vi "SectorOverlay.vi"(0 "Min z":dbl format="%.2f", 1 "Abs?":bool=TRUE, 2 "Interp Mode":i32=1, 5 "Empty Array":dbl[][](array[numeric]) format="%.2f", 7 "x Scaled":dbl[][](array[numeric]) format="%.2f", 9 "y Scaled":dbl[][](array[numeric]) format="%.2f", 11 "z values":dbl[][](array[numeric]) format="%.2f", 12 "Smooth factor":i32=3) -> (10 "raw sector out":dbl[][](array[numeric]) format="%.2f")   [LabVIEW 2022 SP3]
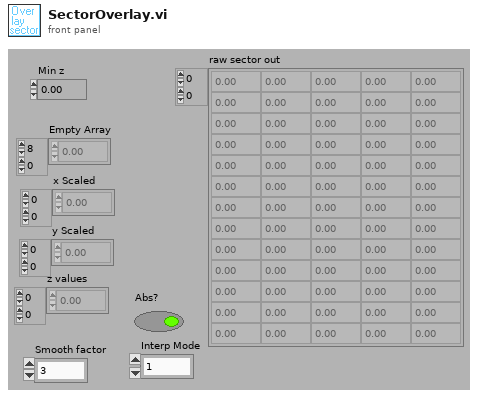
[diagram p1: front panel]
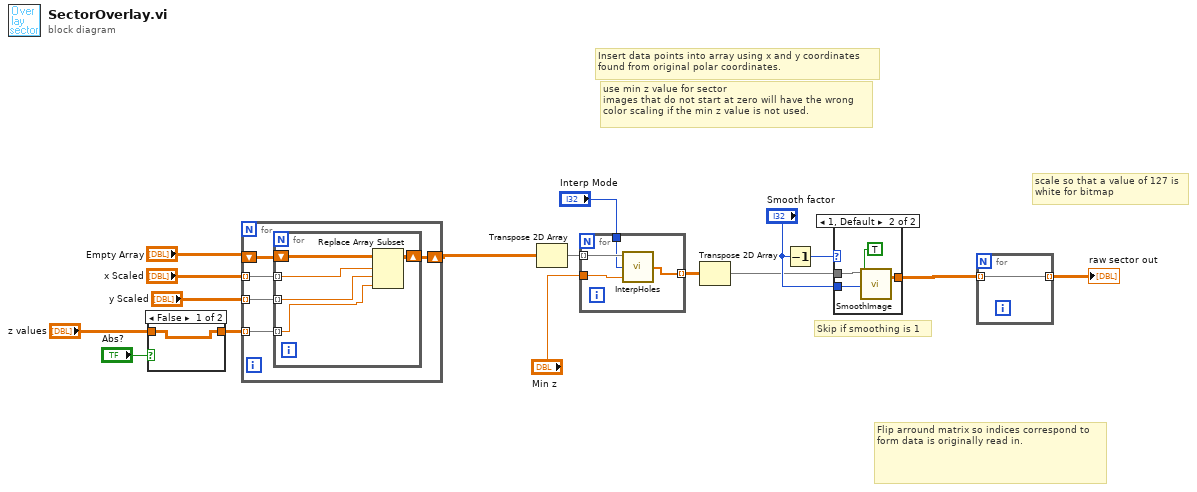
[diagram p0: block diagram]
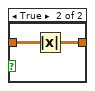
[diagram p2: hidden frame]
diagram:
  # "Skip if smoothing is 1"
  # "use min z value for sector\nimages that do not start at zero will have the wrong\ncolor scaling if the min z value is not used."
  # "Insert data points into array using x and y coordinates\nfound from original polar coordinates."
  # "Flip arround matrix so indices correspond to form data is originally read in."
  # "scale so that a value of 127 is \nwhite for bitmap"
  n1 = case shown="False" "Abs?" {
    tunnel: "z values" -> [w17 w19]
    tunnel: [w17 w18] -> w7
    frame False {
    }
    frame True {
      n2 = Absolute Value(x=w19) -> (abs(x)=w18:dbl[][])
    }
  }
  n3 = for {
    tunnel: w7 -> [w24] mode=indexing
    shift-right: [w22] -> w9
    shift-left: "Empty Array" -> [w23]
    tunnel: "x Scaled" -> [w21] mode=indexing
    tunnel: "y Scaled" -> [w20] mode=indexing
    n4 = for {
      tunnel: w24 -> [w25] mode=indexing
      shift-right: [w28] -> w22
      shift-left: w23 -> [w29]
      tunnel: w21 -> [w27] mode=indexing
      tunnel: w20 -> [w26] mode=indexing
      n5 = Replace Array Subset(array=w29, new element=w25, index (row)=w27, index (col)=w26) -> (w28:dbl[][])
    }
  }
  n6 = Transpose 2D Array(2D array=w9) -> (transposed array=w3:dbl[][])
  n7 = for {
    tunnel: w3 -> [w33] mode=indexing
    tunnel: "Min z" -> [w32]
    tunnel: [w31] -> w2 mode=indexing
    tunnel: "Interp Mode" -> [w30]
    n8 = call "InterpHoles.vi"("min value"=w32, "Interp Mode"=w30, "input array"=w33) -> ("output array"=w31:dbl[])
  }
  n9 = Transpose 2D Array(2D array=w2) -> (transposed array=w6:dbl[][])
  n10 = Decrement(x="Smooth factor") -> (x-1=w15:i32)
  n11 = case shown="1, Default" w15 {
    tunnel: [w34 w36] -> w12
    tunnel: "Smooth factor" -> [_ w37]
    tunnel: w6 -> [w34 w35]
    frame 0 {
    }
    frame 1, Default {
      n12 = call "SmoothImage.vi"("sector array in"=w35, "Override min fill?"=TRUE, "Av size"=w37) -> ("Smoothed Sector w/Ave"=w36:cdb[][])  [unwired: 1 in, 3 out]
    }
  }
  n13 = for {
    tunnel: w12 -> [w39] mode=indexing
    tunnel: [w39] -> w13 mode=indexing
  }
  "raw sector out" <- w13
